vi "Ej 20 Cinta.vi"() -> ()   [LabVIEW 2020]
panel:
  in  "Knob":dbl(knob) scale=0.0..10.0
  out "Slide":dbl(slide) scale=0.0..10.0
  out "Boolean 2":bool
  in  "Boolean":bool
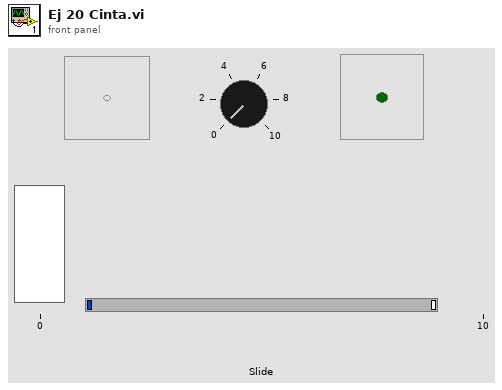
[diagram p1: front panel]
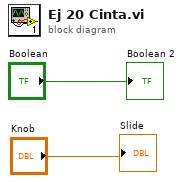
[diagram p0: block diagram]
diagram:
  "Boolean 2" <- "Boolean"
  "Slide" <- "Knob"
